vi "Seq Dialog Set RSLinx Tag String.vi"(8 "Segment Data":T3) -> (0 "Step Hisitory":string[](array[string]), 2 "Segment Data 2":T3)   [LabVIEW 2018]
uses:
  type defs/plc path and tag.ctl
  <vilib>/Platform/dataskt.llb/DataSocket Reference Type.ctl
  type defs/Sequence Info.ctl
  type defs/RSLinx String Cluster.ctl
panel:
  in  "Data String":string
  in  "Tag String":T1={"Tag Name"="S060.PXI.Signals.PlltData.SN", "Network Path"="172.15.51.1,1,0", "use opc"=FALSE, "DataSocket Reference"={"CWDSLib._DCWDataSocket"=refnum, "CWDSLib._DCWData"=refnum, "OnDataUpdated"=0, "OnStatusUpdated"=0}} {"DataSocket Reference"."OnStatusUpdated" format="%.0x"; "DataSocket Reference"."OnDataUpdated" format="%.0x"}
  out "Name":string="Pre Run Station - Glass - Vent Open"
  in  "Description":string
  in  "Save":bool
  in  "Cancel":bool
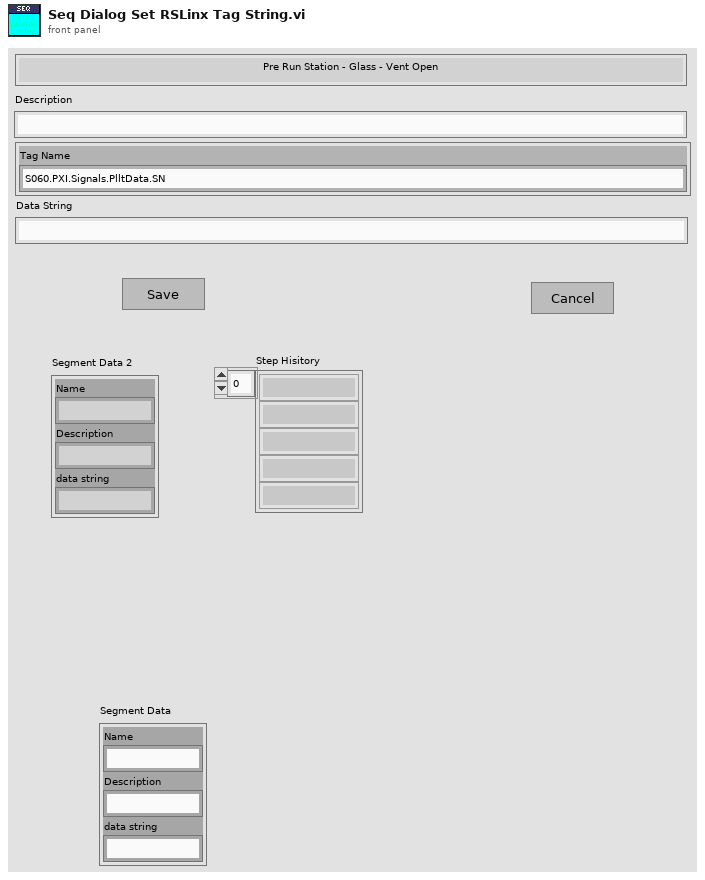
[diagram p1: front panel]
types:
  T1 = typedef "plc path and tag.ctl" = cluster{"Tag Name":string, "Network Path":string, "use opc":bool, "DataSocket Reference":T2}
  T2 = typedef "DataSocket Reference Type.ctl" = cluster{"CWDSLib._DCWDataSocket":refnum<k7>, "CWDSLib._DCWData":refnum<k7>, "OnDataUpdated":u32, "OnStatusUpdated":u32}
  T3 = typedef "Sequence Info.ctl" = cluster{"Name":string, "Description":string, "data string":string}
  T4 = typedef "RSLinx String Cluster.ctl" = cluster{"Data String":string, "PLC Path and Tag":T1, "Error No.":u16, "timeout (ms)":i32}
  T5 = cluster{"Segment Data":T3, "Old Data":string, "New Data":string, "RSLinx String Cluster":T4}
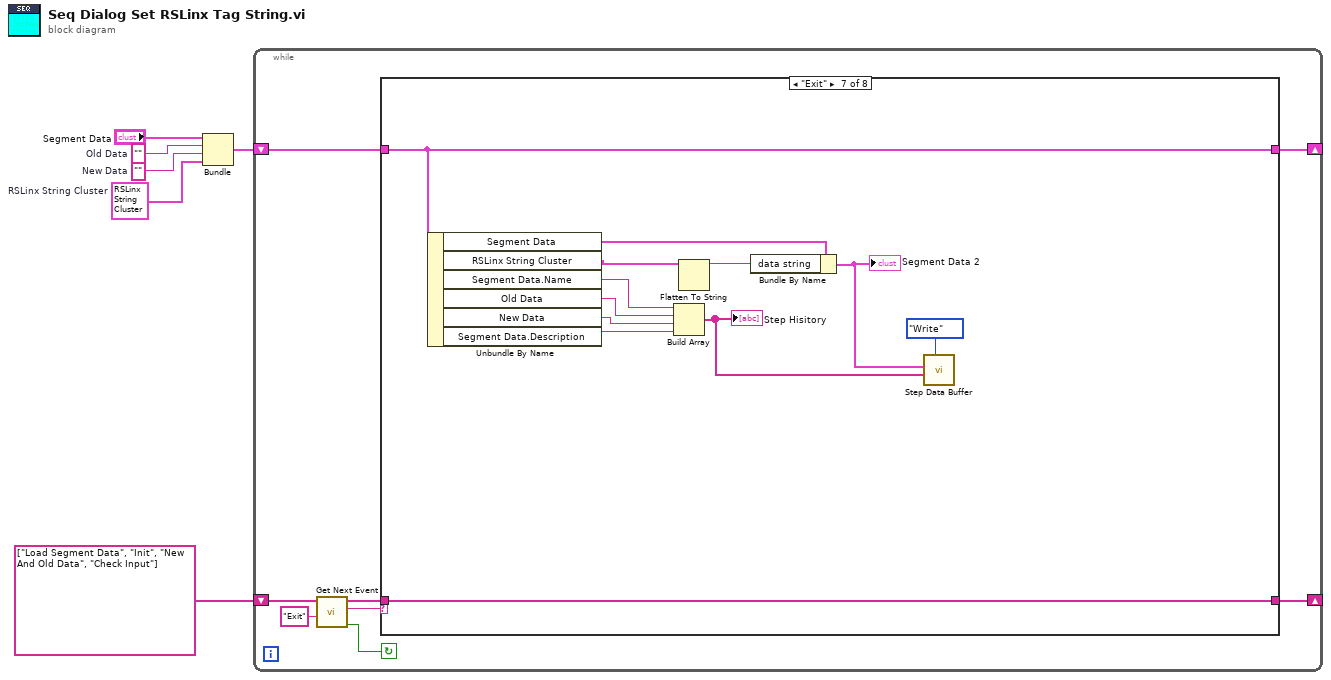
[diagram p0: block diagram]
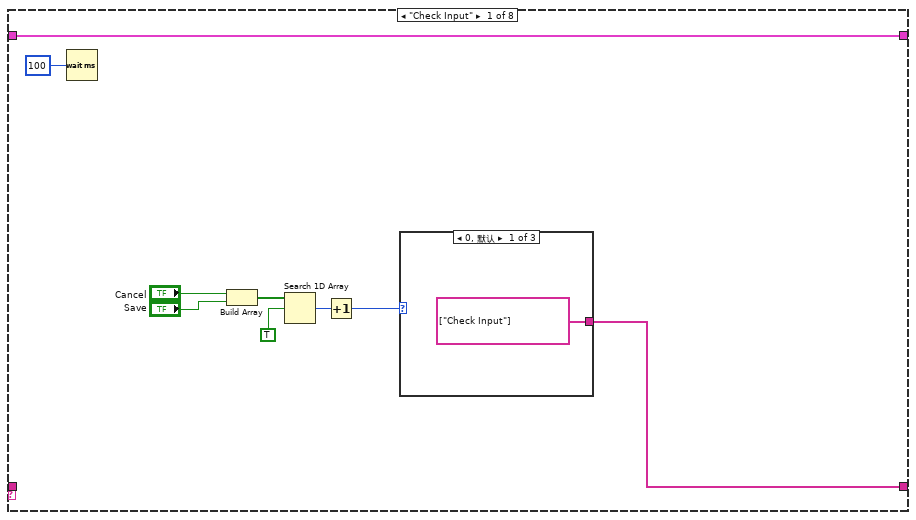
[diagram p2: hidden frame]
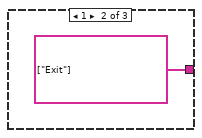
[diagram p3: hidden frame]
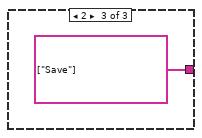
[diagram p4: hidden frame]
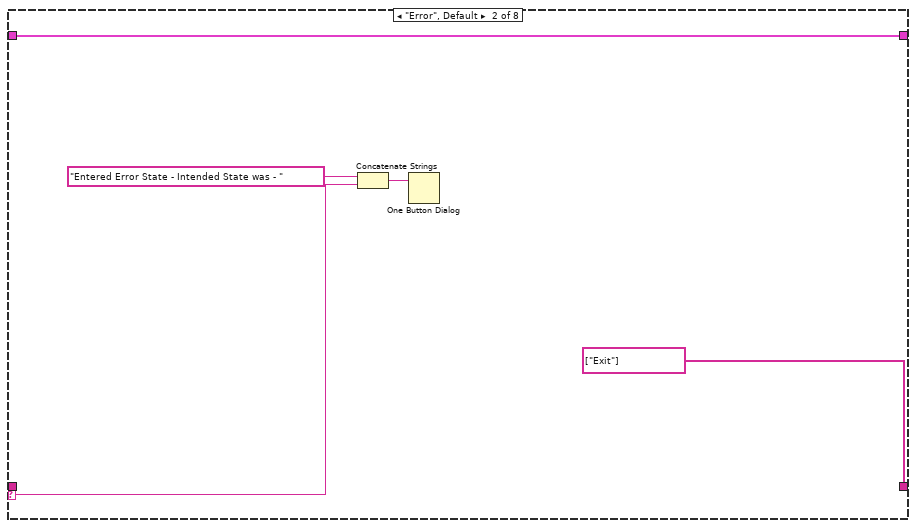
[diagram p5: hidden frame]
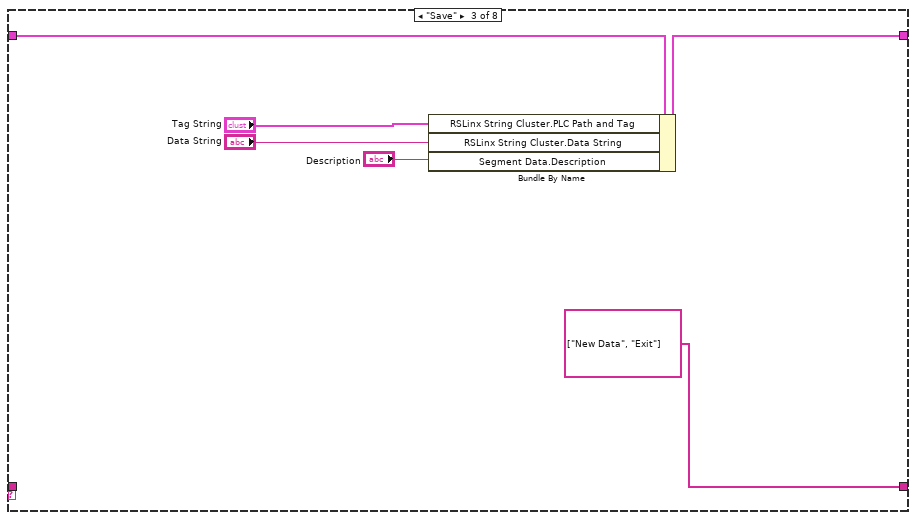
[diagram p6: hidden frame]
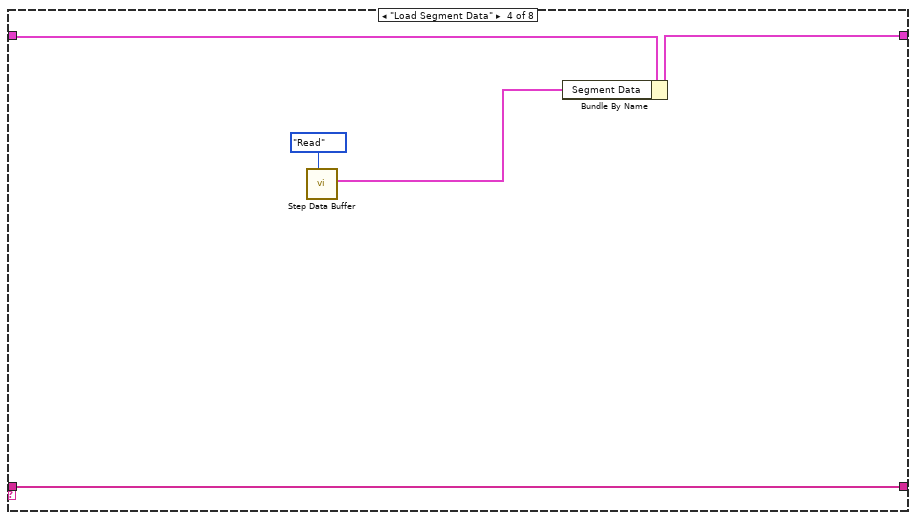
[diagram p7: hidden frame]
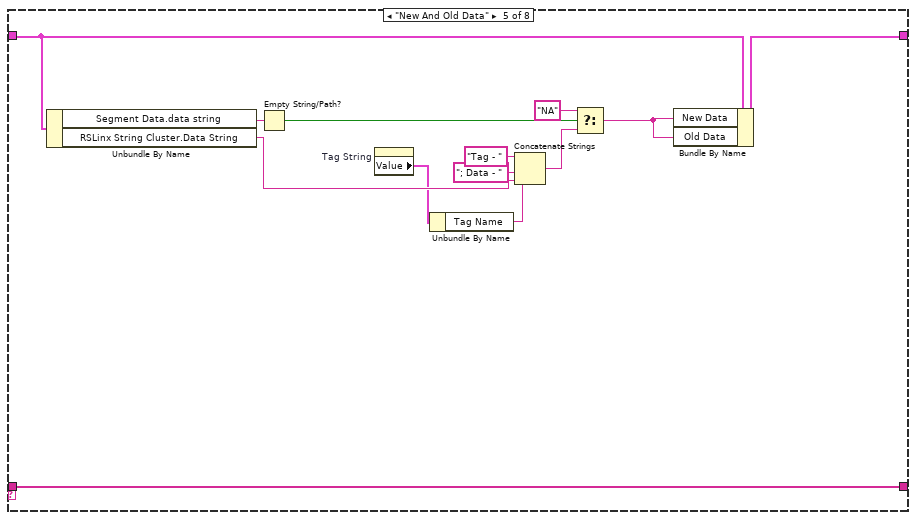
[diagram p8: hidden frame]
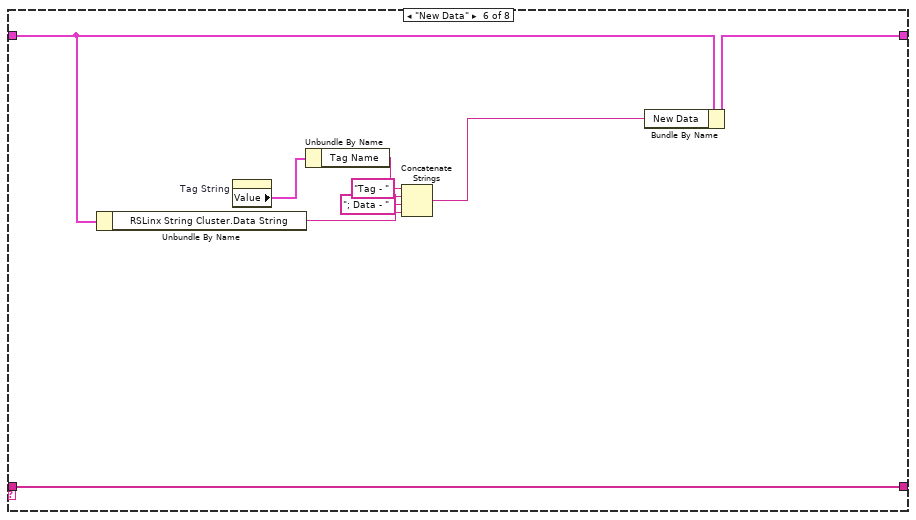
[diagram p9: hidden frame]
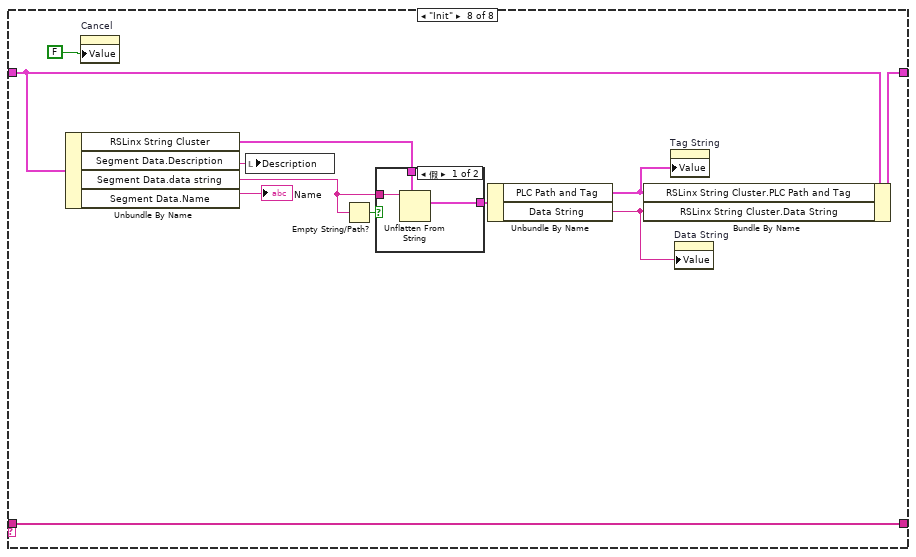
[diagram p10: hidden frame]
diagram:
  w1 = T4 {"Data String"="", "PLC Path and Tag"={"Tag Name"="", "Network Path"="", "use opc"=FALSE, "DataSocket Reference"={"CWDSLib._DCWDataSocket"=refnum, "CWDSLib._DCWData"=refnum, "OnDataUpdated"=0, "OnStatusUpdated"=0}}, "Error No."=0, "timeout (ms)"=0}  # RSLinx String Cluster
  w3 = ""  # New Data
  w4 = ""  # Old Data
  n1 = Bundle("Segment Data"="Segment Data", "Old Data"=w4, "New Data"=w3, "RSLinx String Cluster"=w1) -> (w6:T5)  [unwired: 1 in]
  n2 = while {
    shift-right: [w12] -> _
    shift-left: string[] ["Load Segment Data", "Init", "New And Old Data", "Check Input"] ("Event queue out") -> [w11]
    shift-right: [w7] -> _
    shift-left: w6 -> [w8]
    stop <- w10 continue-if-true
    n3 = call "Get Next Event.vi"("Exit Event"="Exit", "event queue in"=w11) -> ("Condition (Exit:F)"=w10:bool, "next event"=w14:string, "event queue out"=w13:string[])  [unwired: 3 in]
    n4 = case shown="\"Exit\"" w14 {
      selector: w14 -> [_ w29 _ _ _ _ _ _]
      tunnel: w13 -> [_ _ _ w38 w49 w64 w76 w88]
      tunnel: [w17 string[] ["Exit"] ("event queue out") string[] ["New Data", "Exit"] ("Event queue out") w38 w49 w64 w76 w88] -> w12
      tunnel: w8 -> [w22 w27 w36 w40 w51 w63 w75 w83]
      tunnel: [w22 w27 w37 w39 w50 w62 w75 w79] -> w7
      frame "Check Input" {
        n5 = Wait (ms)(milliseconds to wait=u32 100) -> ()  [unwired: 1 out]
        n6 = Build Array("Cancel", "Save") -> (w19:bool[])
        n7 = Search 1D Array(1D array=w19, element=TRUE) -> (index of element=w20:i32)  [unwired: 1 in]
        n8 = Increment(x=w20) -> (x+1=w21:i32)
        n9 = case shown="0, 默认" w21 {
          tunnel: [string[] ["Check Input"] ("Events to Insert") string[] ["Exit"] ("Events to Insert") string[] ["Save"] ("Events to Insert")] -> w17
          frame 0, Default {
          }
          frame 1 {
          }
          frame 2 {
          }
        }
      }
      frame "Error", Default {
        n10 = Concatenate Strings("Entered Error State - Intended State was - " ("string"), w29) -> (w31:string)
        n11 = One Button Dialog(message=w31) -> ()  [unwired: 1 in, 1 out]
      }
      frame "Save" {
        n12 = Bundle By Name(cluster=w36, "RSLinx String Cluster.PLC Path and Tag"="Tag String", "RSLinx String Cluster.Data String"="Data String", "Segment Data.Description"="Description") -> (w37:T5)
      }
      frame "Load Segment Data" {
        n13 = call "Step Data Buffer.vi"("Mode"=enum16{"Init", "Read", "Write"}."Read") -> ("Segment Data Out"=w42:T3)  [unwired: 6 in, 4 out]
        n14 = Bundle By Name(cluster=w40, "Segment Data"=w42) -> (w39:T5)
      }
      frame "New And Old Data" {
        n15 = Unbundle By Name(w51) -> ("Segment Data.data string"=w55:string, "RSLinx String Cluster.Data String"=w46:string)
        n16 = Empty String/Path?(string/path=w55) -> (empty?=w52:bool)
        n17 = property on="Tag String" class="Clust (严格)"() -> ("Value"=w44:T1)  [unwired: 2 in, 2 out]
        n18 = Unbundle By Name(w44) -> ("Tag Name"=w43:string)
        n19 = Concatenate Strings("Tag - " ("string"), w43, "; Data - " ("string"), w46) -> (w45:string)
        n20 = Select(t="NA", s=w52, f=w45) -> (s? t:f=w54:string)
        n21 = Bundle By Name(cluster=w51, "New Data"=w54, "Old Data"=w54) -> (w50:T5)
      }
      frame "New Data" {
        n22 = Unbundle By Name(w63) -> ("RSLinx String Cluster.Data String"=w59:string)
        n23 = property on="Tag String" class="Clust (严格)"() -> ("Value"=w57:T1)  [unwired: 2 in, 2 out]
        n24 = Unbundle By Name(w57) -> ("Tag Name"=w56:string)
        n25 = Concatenate Strings("Tag - " ("string"), w56, "; Data - " ("string"), w59) -> (w58:string)
        n26 = Bundle By Name(cluster=w63, "New Data"=w58) -> (w62:T5)
      }
      frame "Exit" {
        n27 = Unbundle By Name(w75) -> ("Segment Data"=w65:T3, "RSLinx String Cluster"=w66:T4, "Segment Data.Name"=w74:string, "Old Data"=w73:string, "New Data"=w72:string, "Segment Data.Description"=w69:string)
        n28 = Build Array(w74, w73, w72, w69) -> (w70:string[])
        "Step Hisitory" <- w70
        n29 = Flatten To String(anything=w66) -> (data string=w68:string)  [unwired: 3 in, 2 out]
        n30 = Bundle By Name(cluster=w65, "data string"=w68) -> (w67:T3)
        "Segment Data 2" <- w67
        n31 = call "Step Data Buffer.vi"("Mode"=enum16{"Init", "Read", "Write"}."Write", "Step Hisitory In"=w70, "Segment Data In"=w67) -> ()  [unwired: 4 in, 5 out]
      }
      frame "Init" {
        n32 = Unbundle By Name(w83) -> ("RSLinx String Cluster"=w84:T4, "Segment Data.Description"=w87:string, "Segment Data.data string"=w81:string, "Segment Data.Name"=→"Name":string)
        n33 = property on="Cancel" class="Bool (严格)"("Value"=FALSE ("Cancel")) -> ()  [unwired: 2 in, 2 out]
        n34 = local write "Description"(w87) -> ()
        n35 = Empty String/Path?(string/path=w81) -> (empty?=w82:bool)
        n36 = case shown="假" w82 {
          tunnel: w81 -> [w91 _]
          tunnel: w84 -> [w90 w92]
          tunnel: [w89 w92] -> w80
          frame False {
            n37 = Unflatten From String(type=w90, binary string=w91) -> (value=w89:T4)  [unwired: 3 in, 2 out]
          }
          frame True {
          }
        }
        n38 = Unbundle By Name(w80) -> ("PLC Path and Tag"=w77:T1, "Data String"=w78:string)
        n39 = Bundle By Name(cluster=w83, "RSLinx String Cluster.PLC Path and Tag"=w77, "RSLinx String Cluster.Data String"=w78) -> (w79:T5)
        n40 = property on="Tag String" class="Clust (严格)"("Value"=w77) -> ()  [unwired: 2 in, 2 out]
        n41 = property on="Data String" class="Str"("Value"=w78) -> ()  [unwired: 2 in, 2 out]
      }
    }
  }
